vi "Read Decimal and Octal Label Tags.vi"(8 "error in":errorcluster, 11 "node in":refnum<k20>) -> (0 "error out":errorcluster, 2 "label (Dec)":u32, 3 "node out":refnum<k20>)   [LabVIEW 2020, in "ARINC 429 Import.lvlib"]
uses:
  ARINC 429 Import.lvlib
  <vilib>/xml/NI_XML.lvlib
  <resource>/objmgr/DOMUserDefRef.rc
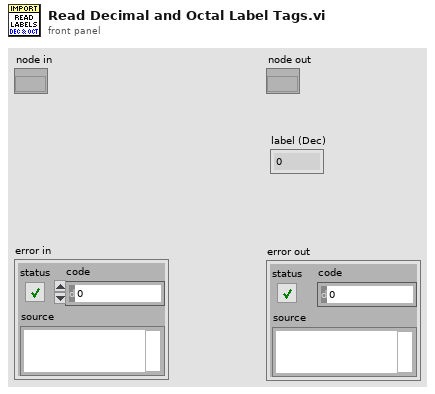
[diagram p1: front panel]
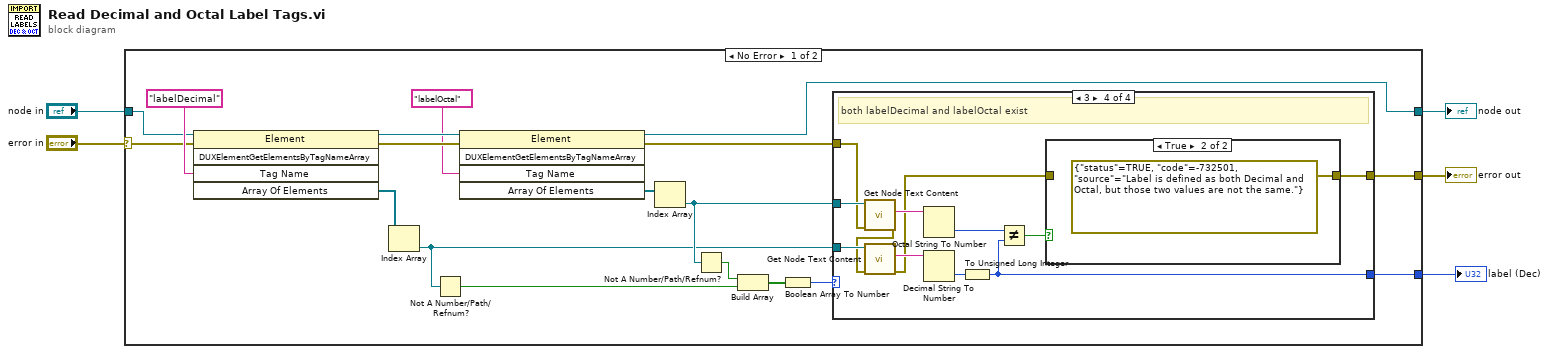
[diagram p0: block diagram]
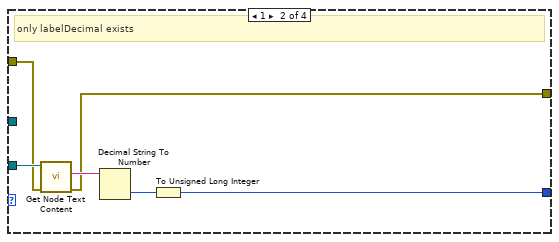
[diagram p3: hidden frame]
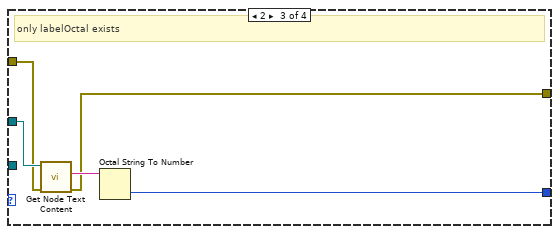
[diagram p4: hidden frame]
diagram:
  n1 = case shown="No Error" "error in" {
    selector: "error in" -> [w8 w51]
    tunnel: [w6 w51] -> w5
    tunnel: "node in" -> [w9 w50]
    tunnel: [w10 w50] -> w3
    tunnel: [w7 _] -> w1
    frame No Error {
      n2 = invoke class="Element" method="DUXElementGetElementsByTagNameArray"(reference=w9, error in=w8, "Tag Name"="labelDecimal") -> (reference out=w15:refnum<k20>, error out=w16:errorcluster, "Array Of Elements"=w12:refnum<k20>[])  [unwired: 2 in, 2 out]
      n3 = Index Array(array=w12) -> (element=w21:refnum<k20>)  [unwired: 1 in]
      n4 = Not A Number/Path/Refnum?(number/path/refnum=w21) -> (NaN/Path/Refnum?=w18:bool)
      n5 = invoke class="Element" method="DUXElementGetElementsByTagNameArray"(reference=w15, error in=w16, "Tag Name"="labelOctal") -> (reference out=w10:refnum<k20>, error out=w23:errorcluster, "Array Of Elements"=w13:refnum<k20>[])  [unwired: 2 in, 2 out]
      n6 = Index Array(array=w13) -> (element=w22:refnum<k20>)  [unwired: 1 in]
      n7 = Not A Number/Path/Refnum?(number/path/refnum=w22) -> (NaN/Path/Refnum?=w17:bool)
      n8 = Build Array(w17, w18) -> (w19:bool[])
      n9 = Boolean Array To Number(Boolean array=w19) -> (number=w20:u32)
      n10 = case shown="3" w20 {
        tunnel: w21 -> [_ w29 _ w44]
        tunnel: w22 -> [_ _ w34 w45]
        tunnel: w23 -> [w24 w28 w33 w43]
        tunnel: [w24 w27 w32 w40] -> w6
        tunnel: [_ w25 w31 w37] -> w7
        frame 0, Default {
          # "neither labelDecimal or labelOctal exist"
        }
        frame 1 {
          # "only labelDecimal exists"
          n11 = call <vilib>:"Get Node Text Content.vi"("error in (no error)"=w28, "node in"=w29) -> ("error out"=w27:errorcluster, "node text"=w30:string)  [unwired: 7 in, 1 out]
          n12 = Decimal String To Number(string=w30) -> (number=w26:i32)  [unwired: 2 in, 1 out]
          n13 = To Unsigned Long Integer(number=w26) -> (unsigned 32bit integer=w25:u32)
        }
        frame 2 {
          # "only labelOctal exists"
          n14 = call <vilib>:"Get Node Text Content.vi"("error in (no error)"=w33, "node in"=w34) -> ("error out"=w32:errorcluster, "node text"=w35:string)  [unwired: 7 in, 1 out]
          n15 = Octal String To Number(4:w35) -> (0:w31:u32)  [unwired: 2 in, 1 out]
        }
        frame 3 {
          # "both labelDecimal and labelOctal exist"
          n16 = call <vilib>:"Get Node Text Content.vi"("error in (no error)"=w43, "node in"=w45) -> ("error out"=w42:errorcluster, "node text"=w46:string)  [unwired: 7 in, 1 out]
          n17 = call <vilib>:"Get Node Text Content.vi"("error in (no error)"=w42, "node in"=w44) -> ("error out"=w39:errorcluster, "node text"=w47:string)  [unwired: 7 in, 1 out]
          n18 = Octal String To Number(4:w46) -> (0:w36:u32)  [unwired: 2 in, 1 out]
          n19 = Decimal String To Number(string=w47) -> (number=w41:i32)  [unwired: 2 in, 1 out]
          n20 = To Unsigned Long Integer(number=w41) -> (unsigned 32bit integer=w37:u32)
          n21 = Not Equal?(x=w36, y=w37) -> (x != y?=w38:bool)
          n22 = case shown="True" w38 {
            tunnel: [w48 errorcluster {"status"=TRUE, "code"=-732501, "source"="Label is defined as both Decimal and Octal, but those two values are not the same."} ("error constant")] -> w40
            tunnel: w39 -> [w48 _]
            frame False {
            }
            frame True {
            }
          }
        }
      }
    }
    frame Error {
    }
  }
  "error out" <- w5
  "node out" <- w3
  "label (Dec)" <- w1
